vi "vipm_BuildDailyVIP.vi"(8 "error in (no error)":errorcluster, 11 "CommandLine":string[](array[string])) -> (0 "error out":errorcluster, 2 "test details":string)   [LabVIEW 2019]
uses:
  <userlib>/_OpenG.lib/file/file.llb/File Exists - Scalar__ogtk.vi
  <userlib>/_OpenG.lib/string/string.llb/Trim Whitespace (String)__ogtk.vi
  <vilib>/JKI/VIPM API/VIPM API_vipm_api.lvlib
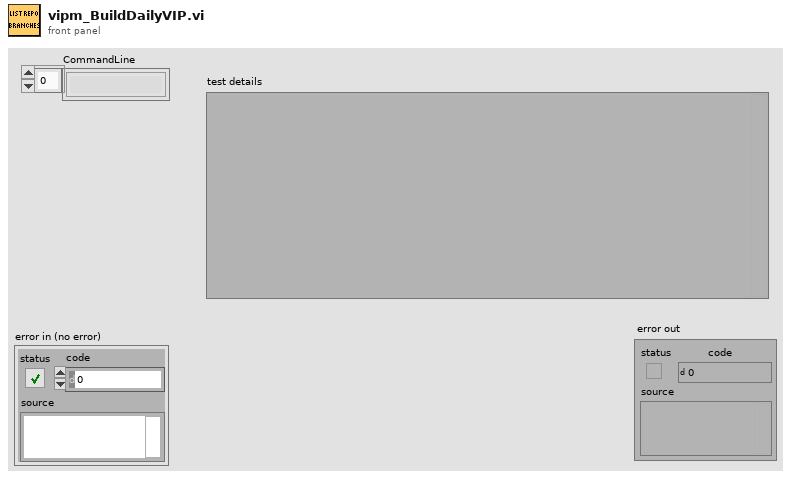
[diagram p1: front panel]
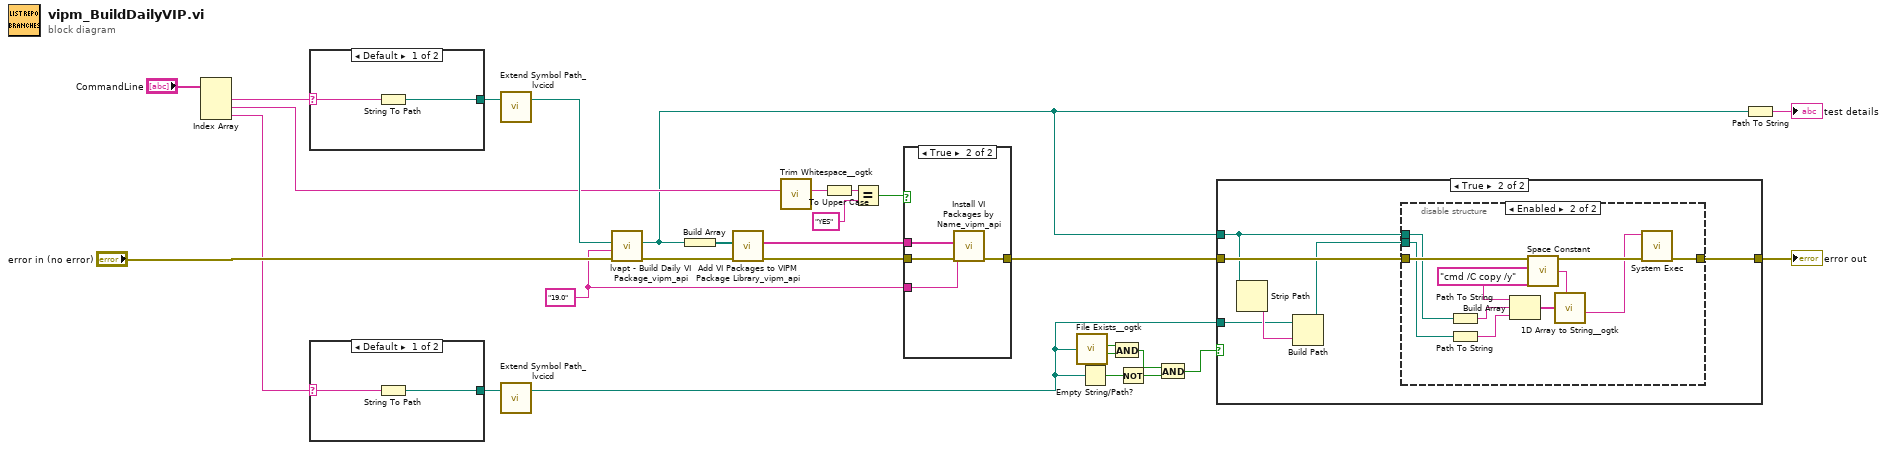
[diagram p0: block diagram]
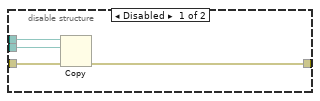
[diagram p3: hidden frame]
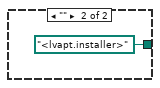
[diagram p4: hidden frame]
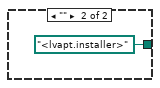
[diagram p6: hidden frame]
diagram:
  w21 = "19.0" ("LabVIEW Version")
  n1 = Index Array(array="CommandLine") -> (element #1=w26:string, element #2=w16:string, element #3=w10:string)  [unwired: 3 in]
  n2 = case shown="Default" w26 {
    selector: w26 -> [w30 _]
    tunnel: [w29 path "<lvapt.installer>"] -> w28
    frame Default {
      n3 = String To Path(string=w30) -> (path=w29:path)
    }
    frame "" {
    }
  }
  n4 = case shown="Default" w10 {
    selector: w10 -> [w33 _]
    tunnel: [w32 path "<lvapt.installer>"] -> w11
    frame Default {
      n5 = String To Path(string=w33) -> (path=w32:path)
    }
    frame "" {
    }
  }
  n6 = call "Extend Symbol Path_lvcicd.vi"("Symbol Path"=w28) -> ("Resolved Path"=w25:path)  [unwired: 2 in]
  n7 = call "Extend Symbol Path_lvcicd.vi"("Symbol Path"=w11) -> ("Resolved Path"=w5:path)  [unwired: 2 in]
  n8 = call <userlib>:"lvapt - Build Daily VI Package_vipm_api.vi"("error in (no error)"="error in (no error)", "LabVIEW Version"=w21, "vipb"=w25) -> ("error out"=w22:errorcluster, "Build Output"=w8:path)  [unwired: 5 in, 2 out]
  n9 = Build Array(w8) -> (w23:path[])
  n10 = call <vilib>:"Add VI Packages to VIPM Package Library_vipm_api.vi"("error in (no error)"=w22, "Packages to add to VIPM Library (vipc,vip,ogp)"=w23) -> ("error out"=w20:errorcluster, "Package Names Added"=w19:string[])  [unwired: 8 in]
  n11 = call-poly <userlib>:"Trim Whitespace__ogtk.vi"("String in"=w16) -> ("String out"=w13:string)  [unwired: 6 in]
  n12 = To Upper Case(1:w13) -> (0:w14:string)
  n13 = Equal?(x=w14, y="YES") -> (x = y?=w17:bool)
  n14 = case shown="True" w17 {
    tunnel: w20 -> [w35 w39]
    tunnel: [w35 w38] -> w18
    tunnel: w21 -> [_ w37]
    tunnel: w19 -> [_ w36]
    frame False {
    }
    frame True {
      n15 = call <vilib>:"Install VI Packages by Name_vipm_api.vi"("error in (no error)"=w39, "LabVIEW Version"=w37, "Package Names to Install []"=w36) -> ("error out"=w38:errorcluster)  [unwired: 8 in]
    }
  }
  n16 = call-poly <userlib>:"File Exists__ogtk.vi"("file path"=w5) -> ("is directory"=w7:bool, "exists"=w6:bool)  [unwired: 6 in]
  n17 = Empty String/Path?(string/path=w5) -> (empty?=w4:bool)
  n18 = And(x=w7, y=w6) -> (x .and. y?=w3:bool)
  n19 = Not(x=w4) -> (.not. x?=w1:bool)
  n20 = And(x=w3, y=w1) -> (x .and. y?=w2:bool)
  n21 = case shown="True" w2 {
    tunnel: w18 -> [w40 w46]
    tunnel: [w40 w45] -> w9
    tunnel: w8 -> [_ w43]
    tunnel: w5 -> [_ w41]
    frame False {
    }
    frame True {
      n22 = Strip Path(path=w43) -> (name=w42:string)  [unwired: 1 out]
      n23 = Build Path(base path=w41, name or relative path=w42) -> (appended path=w44:path)
      n24 = disable-structure shown="Enabled" {
        disable-tunnel: w46 -> [w50 w59]
        disable-tunnel: [w49 w60] -> w45
        disable-tunnel: w44 -> [w48 w57]
        disable-tunnel: w43 -> [w47 w58]
        frame Disabled {
          n25 = Copy(8:w50, 10:w48, 11:w47) -> (0:w49:errorcluster)  [unwired: 2 in, 2 out]
        }
        frame Enabled {
          n26 = Path To String(path=w58) -> (string=w55:string)
          n27 = Path To String(path=w57) -> (string=w54:string)
          n28 = Build Array("cmd /C copy /y" ("name"), w55, w54) -> (w53:string[])
          n29 = call <vilib>:"Space Constant.vi"() -> ("String"=w52:string)
          n30 = call <userlib>:"1D Array to String__ogtk.vi"("delimiter (Tab)"=w52, "Array of Strings"=w53) -> ("delimited string"=w51:string)  [unwired: 9 in]
          n31 = call <vilib>:"System Exec.vi"("error in (no error)"=w59, "command line"=w51) -> ("error out"=w60:errorcluster)  [unwired: 6 in, 3 out]
        }
      }
    }
  }
  "error out" <- w9
  n32 = Path To String(path=w8) -> (string=→"test details":string)
